vi "DDPoseEst2_AbsPoseEst_Work.vi"(5 "Track Width FT":dbl, 6 "InitialPose FT":T1={"TRANSLATION"={"X"=0.0, "Y"=0.0}, "ROTATION"={"VALUE"=0.0, "COS"=1.0, "SIN"=0.0}} {"ROTATION"."SIN" format="%13.4f"; "ROTATION"."COS" format="%13.4f"; "ROTATION"."VALUE" format="%13.4f"; "TRANSLATION"."Y" format="%14.3f"; "TRANSLATION"."X" format="%14.3f"}, 8 "Init":bool, 9 "Gyro Continous\n (inc counterclockwise)\nDEG":dbl, 10 "Right Distance FT":dbl, 11 "Left Distance FT":dbl) -> (4 "Odometry Pose Meters":T1={"TRANSLATION"={"X"=0.0, "Y"=0.0}, "ROTATION"={"VALUE"=0.0, "COS"=1.0, "SIN"=0.0}} {"ROTATION"."SIN" format="%13.4f"; "ROTATION"."COS" format="%13.4f"; "ROTATION"."VALUE" format="%13.4f"; "TRANSLATION"."Y" format="%14.3f"; "TRANSLATION"."X" format="%14.3f"})   [LabVIEW 2019]
uses:
  <vilib>/Rock Robotics/WPI/ThirdParty/JAS_Junk/TrajLib/TypeDef/POSE2D.ctl
  <vilib>/Rock Robotics/WPI/ThirdParty/JAS_Junk/TrajLib/TypeDef/TRANSLATION2D.ctl
  <vilib>/Rock Robotics/WPI/ThirdParty/JAS_Junk/TrajLib/TypeDef/ROTATION2D.ctl
  <vilib>/Rock Robotics/WPI/ThirdParty/JAS_Junk/TrajLib/VI/Util_GetTime_U32.vi
  <vilib>/Rock Robotics/WPI/ThirdParty/JAS_Junk/TrajLib/Rotation2d_CreateAngle.vi
  <vilib>/Rock Robotics/WPI/ThirdParty/JAS_Junk/TrajLib/Translation2d_Create.vi
  <vilib>/Rock Robotics/WPI/ThirdParty/JAS_Junk/TrajLib/VI/Util_GetTime_U64.vi
  <vilib>/Rock Robotics/WPI/ThirdParty/JAS_Junk/TrajLib/Trajectory_Library.lvlib
panel:
  in  "Add Vision Meas":bool
  in  "visionRobotPose":T1={"TRANSLATION"={"X"=0.0, "Y"=0.0}, "ROTATION"={"VALUE"=0.0, "COS"=1.0, "SIN"=0.0}} {"ROTATION"."SIN" format="%13.4f"; "ROTATION"."COS" format="%13.4f"; "ROTATION"."VALUE" format="%13.4f"; "TRANSLATION"."Y" format="%14.3f"; "TRANSLATION"."X" format="%14.3f"}
  in  "Vision TImeStamp_Seconds":dbl=0.02
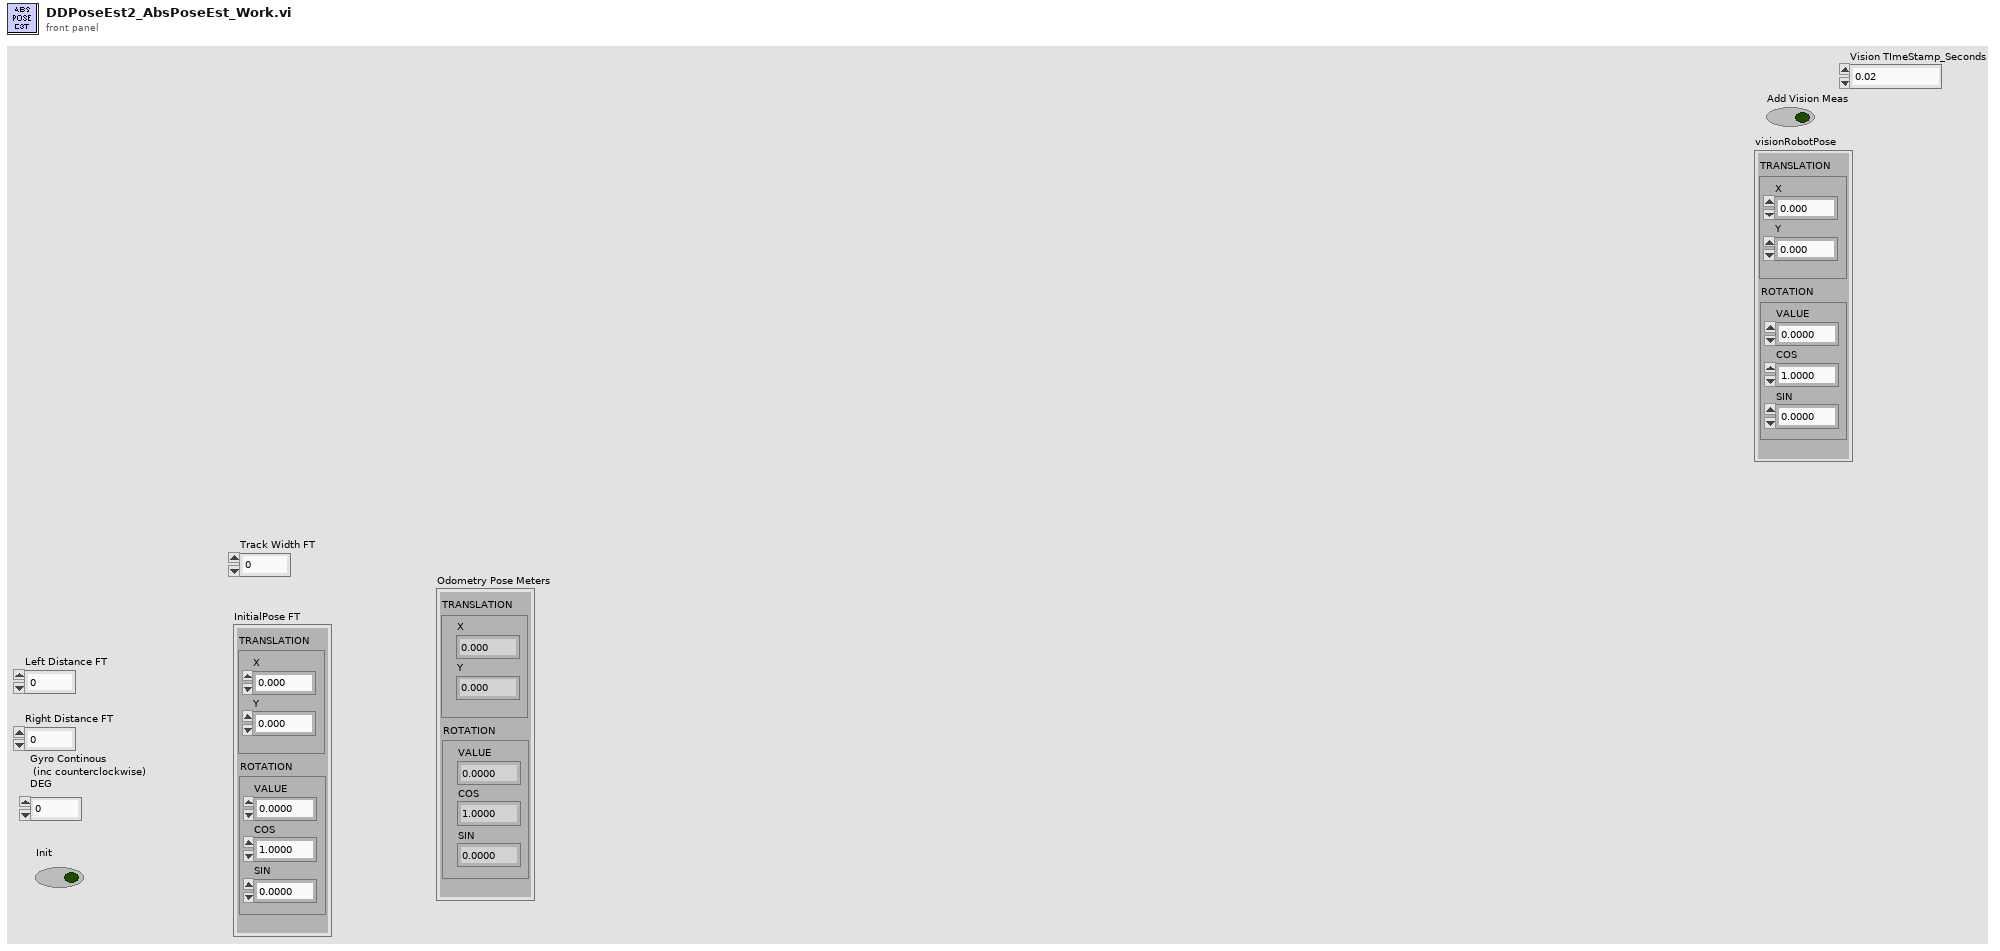
[diagram p1: front panel]
types:
  T1 = typedef "Trajectory_Library.lvlib/POSE2D.ctl" = cluster{"TRANSLATION":T2, "ROTATION":T3}
  T2 = typedef "Trajectory_Library.lvlib/TRANSLATION2D.ctl" = cluster{"X":dbl, "Y":dbl}
  T3 = typedef "Trajectory_Library.lvlib/ROTATION2D.ctl" = cluster{"VALUE":dbl, "COS":dbl, "SIN":dbl}
  T4 = typedef "Trajectory_Library.lvlib/DIFF_DRIVE_POSE_EST2_CONFIG.ctl" = cluster{"TrackWidth_Meters":dbl, "Odom X std dev M":dbl, "Odom Y std dev M":dbl, "Odom Heading std dev Rad":dbl, "Vision X std dev M":dbl, "Vision Y std dev M":dbl, "Vision Heading std dev Rad":dbl}
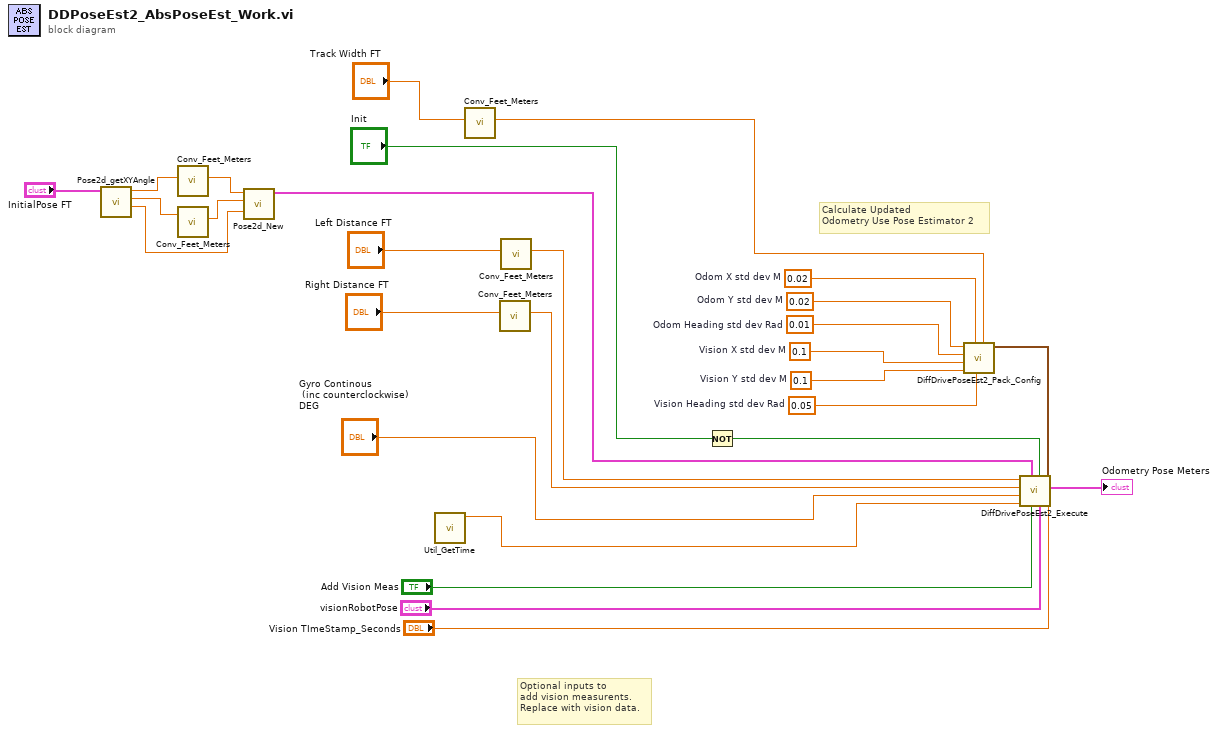
[diagram p0: block diagram]
diagram:
  w19 = 0.02  # Odom Y std dev M
  w20 = 0.01  # Odom Heading std dev Rad
  w21 = 0.1  # Vision X std dev M
  w22 = 0.1  # Vision Y std dev M
  w23 = 0.02  # Odom X std dev M
  w24 = 0.05  # Vision Heading std dev Rad
  # "Optional inputs to\nadd vision measurents.\nReplace with vision data."
  # "Calculate Updated\nOdometry Use Pose Estimator 2"
  n1 = call <vilib>:"Pose2d_getXYAngle.vi"("in POSE"="InitialPose FT") -> ("Angle"=w2:dbl, "Y"=w5:dbl, "X"=w6:dbl)  [unwired: 8 in]
  n2 = call <vilib>:"Conv_Feet_Meters.vi"("Feet"=w6) -> ("Meters"=w4:dbl)  [unwired: 10 in]
  n3 = call <vilib>:"Conv_Feet_Meters.vi"("Feet"=w5) -> ("Meters"=w3:dbl)  [unwired: 10 in]
  n4 = call <vilib>:"Pose2d_New.vi"("Heading"=w2, "Y"=w3, "X"=w4) -> ("out POSe"=w1:T1)  [unwired: 8 in]
  n5 = call <vilib>:"Util_GetTime.vi"() -> ("FPGA_Time_Seconds"=w11:dbl)  [unwired: 9 in, 2 out]
  n6 = call <vilib>:"Conv_Feet_Meters.vi"("Feet"="Track Width FT") -> ("Meters"=w15:dbl)  [unwired: 10 in]
  n7 = call <vilib>:"Conv_Feet_Meters.vi"("Feet"="Right Distance FT") -> ("Meters"=w12:dbl)  [unwired: 10 in]
  n8 = call <vilib>:"Conv_Feet_Meters.vi"("Feet"="Left Distance FT") -> ("Meters"=w9:dbl)  [unwired: 10 in]
  n9 = Not(x="Init") -> (.not. x?=w14:bool)
  n10 = call <vilib>:"DiffDrivePoseEst2_Pack_Config.vi"("TrackWidth_Meters"=w15, "Vision Heading std dev Rad"=w24, "Odom X std dev M"=w23, "Vision Y std dev M"=w22, "Vision X std dev M"=w21, "Odom Heading std dev Rad"=w20, "Odom Y std dev M"=w19) -> ("DiffPoseEst2Config"=w25:T4)  [unwired: 4 in]
  n11 = call <vilib>:"DiffDrivePoseEst2_Execute.vi"("Vision TImeStamp_Seconds"="Vision TImeStamp_Seconds", "DiffPoseEst2Config"=w25, "visionRobotPose"="visionRobotPose", "Game Started"=w14, "Add Vision Meas"="Add Vision Meas", "InitialPose"=w1, "Pass Through Time"=w11, "Gyro Degrees"="Gyro Continous\n (inc counterclockwise)\nDEG", "RightDistance_M"=w12, "LeftDistance_M"=w9) -> ("Estimated Pose"=→"Odometry Pose Meters":T1)  [unwired: 1 out]
